vi "USRP-2945-2955 AoA Detection RX Localization using MUSIC(auto phase calculation using ref signal).vi"() -> ()   [LabVIEW 2015]
uses:
  <instrlib>/niUSRP/niUSRP Timestamp.ctl
  <vilib>/Utility/file.llb/Read Delimited Spreadsheet (DBL).vi
  <instrlib>/niUSRP/niUSRP Configure Time Start Trigger.vi
  <instrlib>/niUSRP/niUSRP Fetch Rx Data (2D CDB).vi
panel:
  in  "Gain":dbl=50.0
  in  "Device Name":refnum<k15>="RIO1"
  out "Antenna Array":dbl[][](array[numeric]) format="%#_4g"
  in  "Carrier Frequency":dbl=900000000.0 format="%#_6p"
  in  "Filter":string(combo)="IIR"
  in  "IQ Rate":dbl=1000000.0 format="%#_6p"
  in  "Threshold\n (See Description)":dbl=0.001
  in  "No. of Samples per Frame":i32=100000
  in  "Samples used":i32=1000
  in  "Stop":bool
  in  "start trigger time":T1={"whole seconds"=1, "fractional seconds"=0.0}
  out "ch3-ch2":dbl[](array[numeric])
  out "ch1-ch2":dbl[](array[numeric])
  out "ch0-ch2":dbl[](array[numeric])
  out "Source Location":dbl[](array[numeric])
  out "Direction":dbl(knob) scale=0.0..180.0
  out "MuSIC spectrum":cluster{"Y":dbl[], "Y":dbl[]}[](graph)
  out "Queue error out":errorcluster
  out "# elements in queue (it should keep 0)":i32
  out "USRP error out":errorcluster
  out "Actual Rx timestamp":T1
  out "Eigenvalue":cdb[][](array[numeric])
  out "Direct wave after phase synchronized":dbl[][](graph) caption="Waveform Graph 1"
  out "Air signal after phase synchronized":dbl[][](graph) caption="Waveform Graph 1"
  out "Direct wave phase before phase synchronized":dbl[][](graph) caption="Waveform Graph 1"
  out "Direct wave phase after phase synchronized":dbl[][](graph) caption="Waveform Graph 1"
  out "Signal phase before phase synchronized":dbl[][](graph) caption="Waveform Graph 1"
  out "Signal phase after phase synchronized":dbl[][](graph) caption="Waveform Graph 1"
  out "The number of sources":i32
  out "Time Processed":dbl
  out "coerced IQ rate":dbl format="%#_6p"
  out "coerced carrier frequency":dbl format="%#_6p"
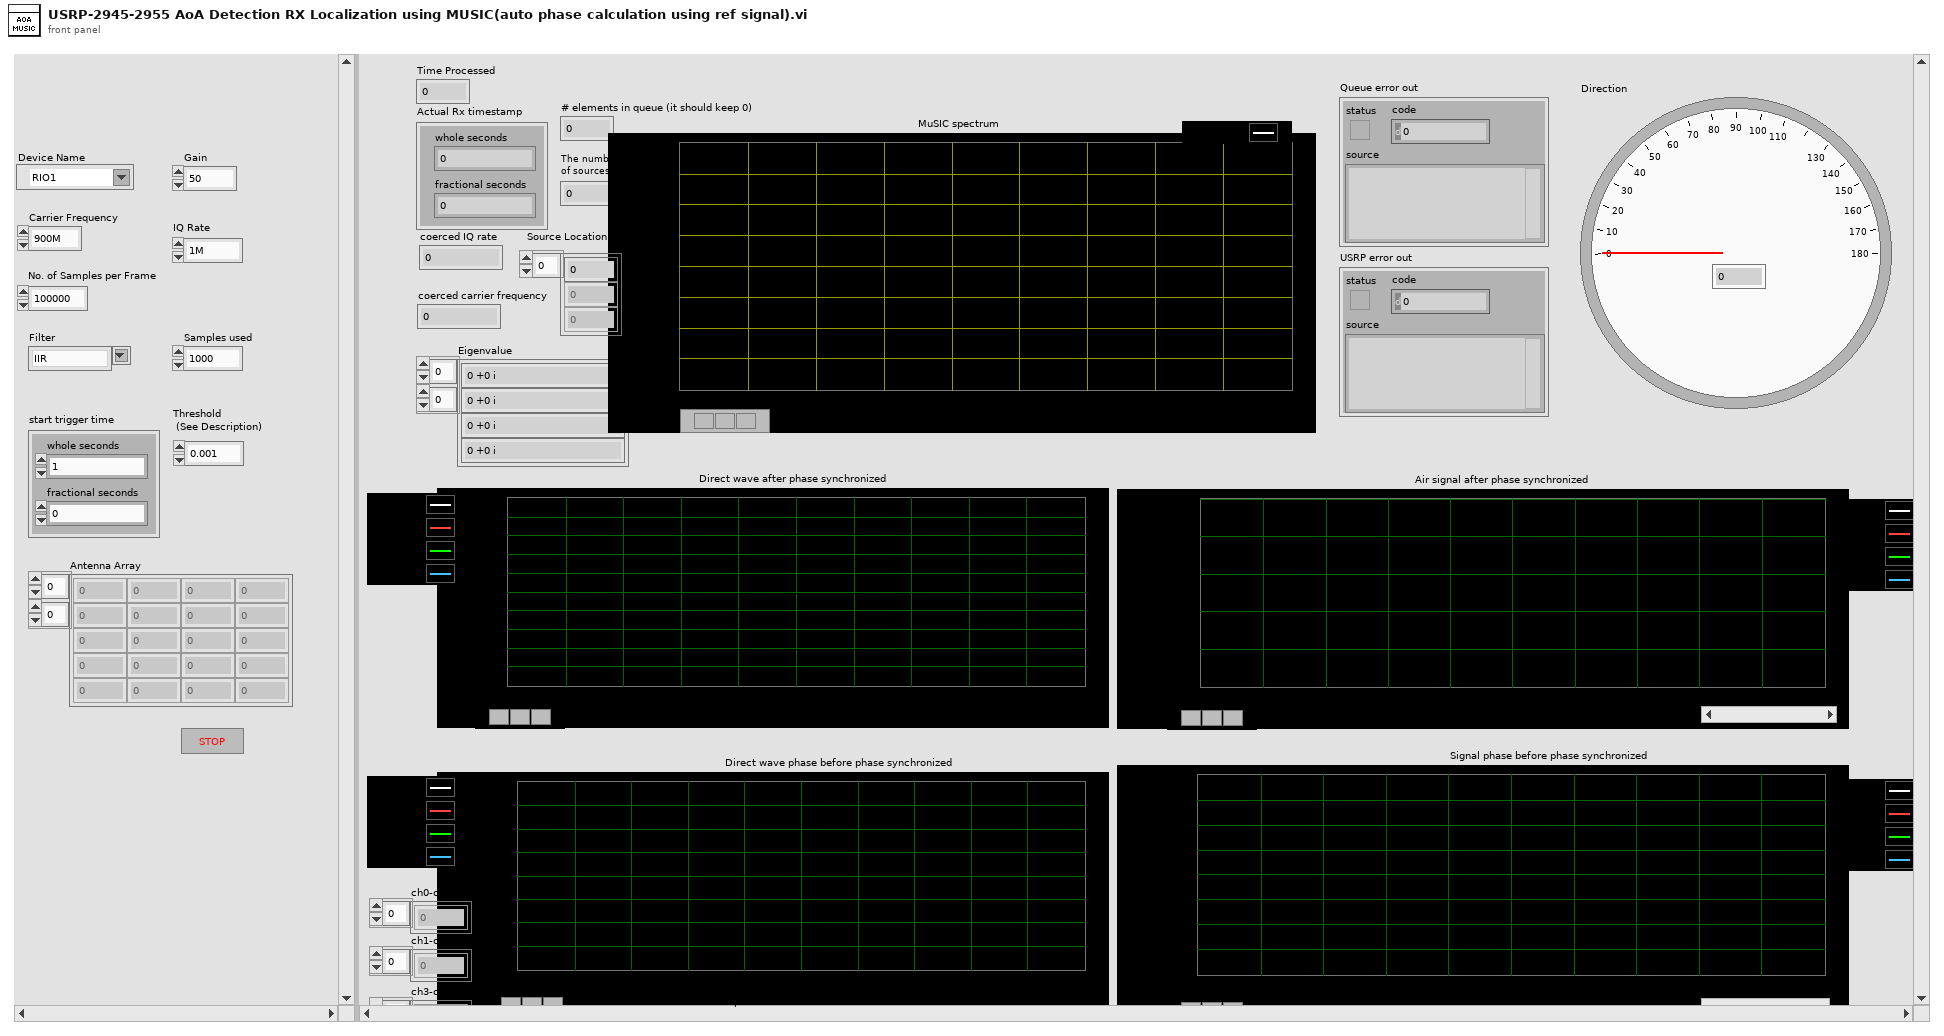
[diagram p1: front panel]
types:
  T1 = typedef "niUSRP Timestamp.ctl" = cluster{"whole seconds":u64, "fractional seconds":dbl}
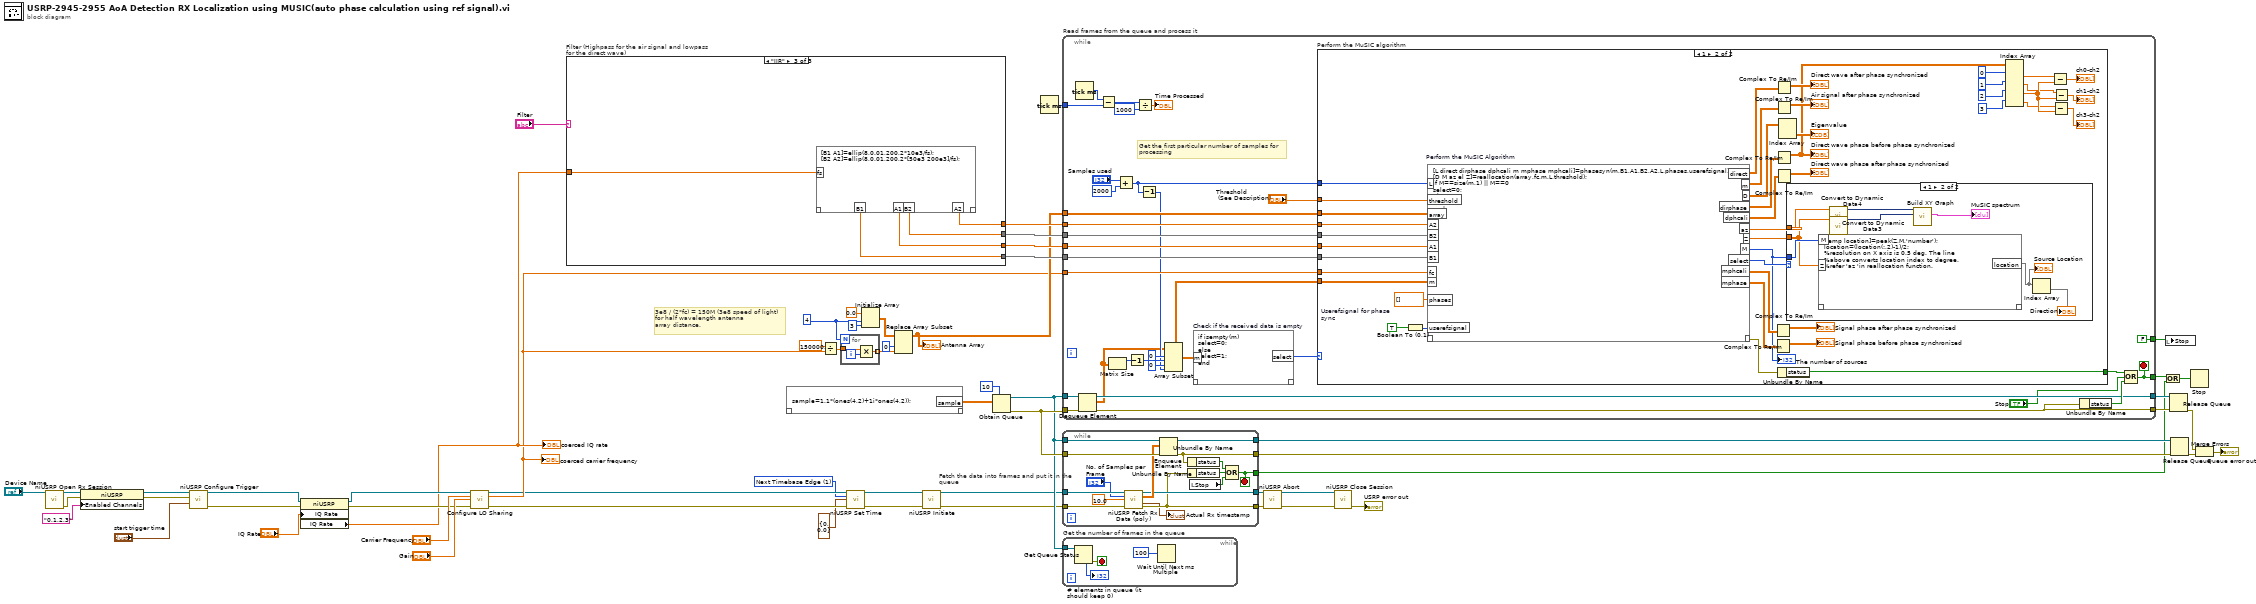
[diagram p0: block diagram]
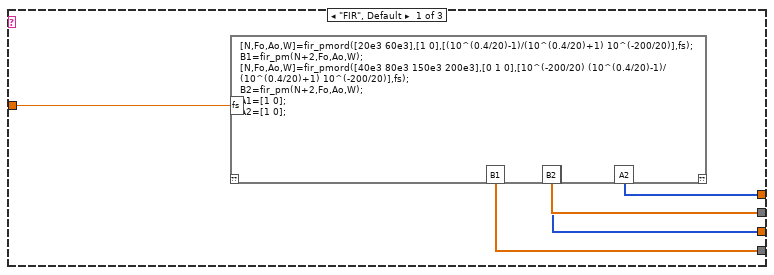
[diagram p2: hidden frame]
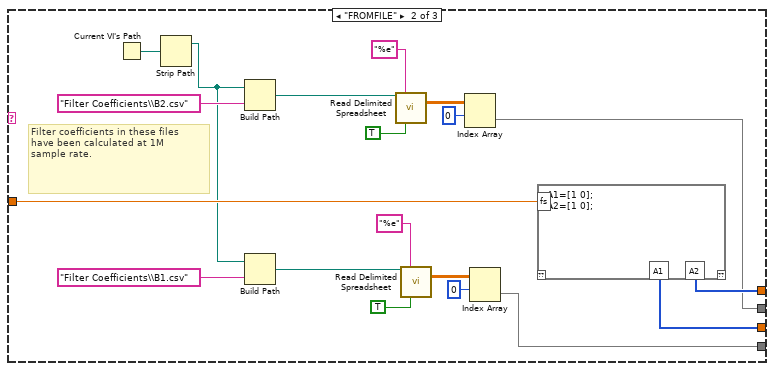
[diagram p3: hidden frame]
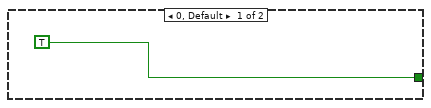
[diagram p4: hidden frame]
diagram:
  w4 = 1 items=["Now", "Next Timebase Edge"] ("apply timestamp")
  w24 = 4
  # "3e8 / (2*fc) = 150M (3e8 speed of light)\nfor half wavelength antenna\narray distance."
  n1 = call <instrlib>:"niUSRP Open Rx Session.vi"("device names"="Device Name") -> ("session handle out"=w22:refnum<k15>, "error out"=w21:errorcluster)  [unwired: 13 in]
  n2 = property class="niUSRP"(reference=w22, error in=w21, "Enabled Channels"="0,1,2,3") -> (reference out=w19:refnum<k15>, error out=w18:errorcluster)
  n3 = call-poly <instrlib>:"niUSRP Configure Trigger.vi"("session handle"=w19, "start trigger time"="start trigger time", "error in (no error)"=w18) -> ("session handle out"=w2:refnum<k15>, "error out"=w1:errorcluster)  [unwired: 11 in]
  n4 = property class="niUSRP"(reference=w2, error in=w1, "IQ Rate"="IQ Rate") -> (reference out=w12:refnum<k15>, error out=w11:errorcluster, "IQ Rate"=w10:dbl)
  "coerced IQ rate" <- w10
  n5 = call "Configure LO Sharing.vi"("reference"=w12, "Carrier Frequency [Hz]"="Carrier Frequency", "Gain"="Gain", "error in"=w11) -> ("reference out"=w6:refnum<k15>, "Coerced Carrier Frequency"=w9:dbl, "error out"=w8:errorcluster)  [unwired: 9 in]
  "coerced carrier frequency" <- w9
  n6 = case "Filter (Highpass for the air signal and lowpass for the direct wave)" shown="\"IIR\"" "Filter" {
    tunnel: [w64 w76 w88] -> w56
    tunnel: [w61 w82 w87] -> w55
    tunnel: [w63 w71 w86] -> w54
    tunnel: [w62 w83 w85] -> w53
    tunnel: w10 -> [w60 w81 w84]
    frame "FIR", Default {
      n7 = mathscript code="[N,Fo,Ao,W]=fir_pmord([20e3 60e3],[1 0],[(10^(0.4/20)-1)/(10^(0.4/20)+1) 10^(-200/20)],fs);\nB1=fir_pm(N+2,Fo,Ao,W);\n[N,Fo,Ao,W]=fir_pmord([40e3 80e3 150e3 200e3],[0 1 0],[10^(-200/20) (10^(0.4/20)-1)/(10^(0.4/20)+1) 10^(-200/20)],fs);\nB2=fir_pm(N+2,Fo,Ao,W);\nA1=[1 0];\nA2=[1 0];"("fs"=w60) -> ("B1"=w64:dbl[], "A1"=w61:i32[], "B2"=w63:dbl[], "A2"=w62:i32[])  [unwired: 1 in, 1 out]
    }
    frame "FROMFILE" {
      # "Filter coefficients in these files\nhave been calculated at 1M\nsample rate."
      n8 = Current VI's Path() -> (path=w70:path)
      n9 = Strip Path(path=w70) -> (stripped path=w66:path)  [unwired: 1 out]
      n10 = Build Path(base path=w66, name or relative path="Filter Coefficients\\B2.csv") -> (appended path=w68:path)
      n11 = Build Path(base path=w66, name or relative path="Filter Coefficients\\B1.csv") -> (appended path=w65:path)
      n12 = call-poly <vilib>:"Read Delimited Spreadsheet.vi"("file path (dialog if empty)"=w68, "format (%.3f)"="%e", "transpose? (F)"=TRUE) -> ("all rows"=w73:dbl[][])  [unwired: 7 in, 5 out]
      n13 = call-poly <vilib>:"Read Delimited Spreadsheet.vi"("file path (dialog if empty)"=w65, "format (%.3f)"="%e", "transpose? (F)"=TRUE) -> ("all rows"=w79:dbl[][])  [unwired: 7 in, 5 out]
      n14 = Index Array(array=w73, index (row)=0) -> (element=w71:dbl[])  [unwired: 1 in]
      n15 = Index Array(array=w79, index (row)=0) -> (element=w76:dbl[])  [unwired: 1 in]
      n16 = mathscript code="A1=[1 0];\nA2=[1 0];"("fs"=w81) -> ("A1"=w82:i32[], "A2"=w83:i32[])  [unwired: 1 in, 1 out]
    }
    frame "IIR" {
      n17 = mathscript code="[B1 A1]=ellip(8,0.01,200,2*10e3/fs);\n[B2 A2]=ellip(8,0.01,200,2*[50e3 200e3]/fs);"("fs"=w84) -> ("A1"=w87:dbl[], "B1"=w88:dbl[], "A2"=w85:dbl[], "B2"=w86:dbl[])  [unwired: 1 in, 1 out]
    }
  }
  n18 = mathscript code="sample=1.1*(ones(4,2)+1i*ones(4,2));"() -> ("sample"=w49:cdb[][])  [unwired: 1 in, 1 out]
  n19 = Divide(x=150000000.0, y=w9) -> (x/y=w32:dbl)
  n20 = for {
    N: w24 -> [_]
    tunnel: w32 -> [w91]
    tunnel: [w90] -> w28 mode=indexing
    i -> [w89]
    n21 = Multiply(x=w91, y=w89) -> (x*y=w90:dbl)
  }
  n22 = call <instrlib>:"niUSRP Set Time.vi"("session handle"=w6, "apply timestamp"=w4, "timestamp"=T1 {"whole seconds"=0, "fractional seconds"=0.0}, "error in (no error)"=w8) -> ("session handle out"=w5:refnum<k15>, "error out"=w7:errorcluster)  [unwired: 10 in]
  n23 = Initialize Array(0.0 ("element"), w24, 3 ("dimension size")) -> (w29:dbl[][])
  n24 = Replace Array Subset(array=w29, new element=w28, index (col)=0 ("disabled index (col)")) -> (w26:dbl[][])  [unwired: 1 in]
  "Antenna Array" <- w26
  n25 = call <instrlib>:"niUSRP Initiate.vi"("session handle"=w5, "error in (no error)"=w7) -> ("session handle out"=w17:refnum<k15>, "error out"=w16:errorcluster)  [unwired: 12 in]
  n26 = Obtain Queue(max queue size (-1, unlimited)=10, element data type=w49) -> (queue out=w38:refnum<queue>, error out=w39:errorcluster)  [unwired: 3 in, 1 out]
  n27 = Tick Count (ms)() -> (millisecond timer value=w51:u32)
  n28 = while "Read frames from the queue and process it" {
    tunnel: w9 -> [w123]
    tunnel: w26 -> [w121]
    tunnel: [w98] -> w42
    tunnel: [w97] -> w41
    tunnel: w56 -> [w120]
    tunnel: w55 -> [w119]
    tunnel: w54 -> [w118]
    tunnel: w53 -> [w117]
    tunnel: w51 -> [w110]
    tunnel: w38 -> [w106]
    tunnel: w39 -> [w105]
    tunnel: [w100] -> w35
    tunnel: [FALSE ("Stop")] -> w25
    stop <- w100 stop-if-true
    # "Get the first particular number of samples for \nprocessing"
    n29 = Tick Count (ms)() -> (millisecond timer value=w111:u32)
    n30 = Dequeue Element(queue=w106, error in (no error)=w105) -> (queue out=w98:refnum<queue>, element=w92:cdb[][], error out=w97:errorcluster)  [unwired: 1 in, 1 out]
    n31 = Subtract(x=w111, y=w110) -> (x-y=w109:u32)
    n32 = Matrix Size(0:w92) -> (1:w104:i32)  [unwired: 1 out]
    n33 = Add(x="Samples used", y=2000) -> (x+y=w95:i32)
    n34 = Decrement(x=w104) -> (x-1=w103:i32)
    n35 = Divide(x=w109, y=1000) -> (x/y=→"Time Processed":dbl)
    n36 = Decrement(x=w95) -> (x-1=w94:i32)
    n37 = Array Subset(array=w92, index (row)=0, length (row)=w103, index (col)=0, length (col)=w94) -> (w114:cdb[][])
    n38 = mathscript code="if isempty(m)\nselect=0;\nelse\nselect=1;\nend" "Check if the received data is empty"("m"=w114) -> ("select"=w99:i32)  [unwired: 1 in, 1 out]
    n39 = case "Perform the MuSIC algorithm" shown="1" w99 {
      tunnel: w123 -> [_ w167]
      tunnel: "Threshold\n (See Description)" -> [_ w164]
      tunnel: w121 -> [_ w163]
      tunnel: [TRUE w145] -> w102
      tunnel: w120 -> [_ w161]
      tunnel: w119 -> [_ w160]
      tunnel: w118 -> [_ w159]
      tunnel: w117 -> [_ w158]
      tunnel: w95 -> [_ w147]
      tunnel: w114 -> [_ w146]
      frame 0, Default {
      }
      frame 1 {
        w138 = TRUE  # Userefsignal for phase  sync
        n40 = Boolean To (0,1)(Boolean=w138) -> (0, 1=w139:i16)
        n41 = mathscript code="[L direct dirphase dphcali m mphase mphcali]=phasesyn(m,B1,A1,B2,A2,L,phases,userefsignal);\n[D M az el Z]=reallocation(array,fc,m,L,threshold);\nif M==size(m,1) || M==0 \nselect=0;\nelse\nselect=1;\nend" "Perform the MuSIC Algorithm"("m"=w146, "fc"=w167, "L"=w147, "array"=w163, "threshold"=w164, "B1"=w161, "A1"=w160, "B2"=w159, "A2"=w158, "phases"=dbl[] [], "userefsignal"=w139) -> ("??"=w155:errorcluster, "D"=w166:cdb[][], "az"=w143:dbl[], "Z"=w142:cdb[], "M"=w140:i32, "m"=w157:cdb[][], "direct"=w148:cdb[][], "dirphase"=w152:dbl[][], "dphcali"=w151:dbl[][], "mphase"=w150:dbl[][], "mphcali"=w149:dbl[][], "select"=w141:i32)  [unwired: 1 in]
        "The number of sources" <- w140
        n42 = Complex To Re/Im(x + iy=w149) -> (x=→"Signal phase after phase synchronized":dbl[][])  [unwired: 1 out]
        n43 = Complex To Re/Im(x + iy=w150) -> (x=→"Signal phase before phase synchronized":dbl[][])  [unwired: 1 out]
        n44 = Complex To Re/Im(x + iy=w148) -> (x=→"Direct wave after phase synchronized":dbl[][])  [unwired: 1 out]
        n45 = Complex To Re/Im(x + iy=w157) -> (x=→"Air signal after phase synchronized":dbl[][])  [unwired: 1 out]
        n46 = Complex To Re/Im(x + iy=w152) -> (x=w137:dbl[][])  [unwired: 1 out]
        "Direct wave phase before phase synchronized" <- w137
        n47 = Complex To Re/Im(x + iy=w151) -> (x=→"Direct wave phase after phase synchronized":dbl[][])  [unwired: 1 out]
        n48 = Unbundle By Name(w155) -> ("status"=w145:bool)
        n49 = Index Array(array=w166) -> (element=→"Eigenvalue":cdb[][])  [unwired: 2 in]
        n50 = case shown="1" w141 {
          tunnel: w143 -> [_ w172]
          tunnel: w142 -> [_ w170]
          tunnel: w140 -> [_ w171]
          frame 0, Default {
          }
          frame 1 {
            n51 = mathscript code="[temp location]=peak(Z,M,'number');\nlocation=(location(:,2)-1)/2;\n%resolution on X axis is 0.5 deg. The line\n%above converts location index to degree.\n%refer 'az 'in reallocation function."("M"=w171, "Z"=w170) -> ("location"=w168)  [unwired: 1 in, 1 out]
            "Source Location" <- w168
            n52 = call "Convert to Dynamic Data4"("Array"=w172) -> ("Dynamic Data Type"=w174:dynamicdata)  [unwired: 3 in]
            n53 = call "Convert to Dynamic Data3"("Array"=w170) -> ("Dynamic Data Type"=w173:dynamicdata)  [unwired: 3 in]
            n54 = call "Build XY Graph"("Y Input"=w173, "X Input"=w174) -> ("XY Graph"=→"MuSIC spectrum":cluster{"Y":dbl[], "Y":dbl[]}[])  [unwired: 3 in, 6 out]
            n55 = Index Array(array=w168) -> (element=→"Direction")  [unwired: 1 in]
          }
        }
        n56 = Index Array(array=w137, index (row) #1=0 ("index (row)"), index (row) #2=1 ("index (row)"), index (row) #3=2 ("index (row)"), index (row) #4=3 ("index (row)")) -> (element #1=w132:dbl[], element #2=w130:dbl[], element #3=w131:dbl[], element #4=w129:dbl[])  [unwired: 4 in]
        n57 = Subtract(x=w132, y=w131) -> (x-y=→"ch0-ch2":dbl[])
        n58 = Subtract(x=w129, y=w131) -> (x-y=→"ch3-ch2":dbl[])
        n59 = Subtract(x=w130, y=w131) -> (x-y=→"ch1-ch2":dbl[])
      }
    }
    n60 = Unbundle By Name(w97) -> ("status"=w101:bool)
    n61 = Compound Arithmetic op=OR(w102, "Stop", w101) -> (w100:bool)
  }
  n62 = while "Fetch the data into frames and put it in the queue" {
    tunnel: w17 -> [w190]
    tunnel: w16 -> [w189]
    tunnel: w38 -> [w188]
    tunnel: w39 -> [w187]
    tunnel: [w185] -> w44
    tunnel: [w182] -> w43
    tunnel: [w184] -> w47
    tunnel: [w183] -> w46
    tunnel: [w176] -> w34
    stop <- w176 stop-if-true
    n63 = call-poly <instrlib>:"niUSRP Fetch Rx Data (poly).vi"("session handle"=w190, "number of samples"="No. of Samples per Frame", "timeout"=10.0, "error in (no error)"=w189) -> ("session handle out"=w184:refnum<k15>, "data"=w186:cdb[][], "timestamp"=→"Actual Rx timestamp":T1, "error out"=w183:errorcluster)  [unwired: 8 in]
    n64 = Enqueue Element(queue=w188, element=w186, error in (no error)=w187) -> (queue out=w185:refnum<queue>, error out=w182:errorcluster)  [unwired: 1 in, 1 out]
    n65 = Unbundle By Name(w182) -> ("status"=w179:bool)
    n66 = Unbundle By Name(w183) -> ("status"=w178:bool)
    n67 = local read "Stop"() -> (w177:bool)
    n68 = Compound Arithmetic op=OR(w179, w178, w177) -> (w176:bool)
  }
  n69 = while "Get the number of frames in the queue" {
    tunnel: w38 -> [w195]
    stop <- w193 stop-if-true
    n70 = Get Queue Status(queue=w195) -> (error out=w193:errorcluster, # elements in queue=→"# elements in queue (it should keep 0)":i32)  [unwired: 2 in, 6 out]
    n71 = Wait Until Next ms Multiple(millisecond multiple=100) -> ()  [unwired: 1 out]
  }
  n72 = call <instrlib>:"niUSRP Abort.vi"("session handle"=w47, "error in (no error)"=w46) -> ("session handle out"=w59:refnum<k15>, "error out"=w58:errorcluster)  [unwired: 12 in]
  n73 = call <instrlib>:"niUSRP Close Session.vi"("session handle"=w59, "error in (no error)"=w58) -> ("error out"=→"USRP error out":errorcluster)  [unwired: 13 in]
  n74 = Or(x=w35, y=w34) -> (x .or. y?=w40:bool)
  n75 = local write "Stop"(w25) -> ()
  n76 = Release Queue(queue=w42, error in (no error)=w41) -> (error out=w36:errorcluster)  [unwired: 1 in, 2 out]
  n77 = Release Queue(queue=w44, error in (no error)=w43) -> (error out=w37:errorcluster)  [unwired: 1 in, 2 out]
  n78 = Stop(stop? (T)=w40) -> ()
  n79 = Merge Errors(w36, w37) -> (→"Queue error out":errorcluster)
